vi "Curtin1_NotesDialog.vi"(11 "Files":T1[](array[typedef])) -> (0 "Color":u32[](array[colorbox]), 2 "removed?":bool, 3 "Array":T1[](array[typedef]))   [LabVIEW 2022 SP3]
uses:
  Curtin1_Label.ctl
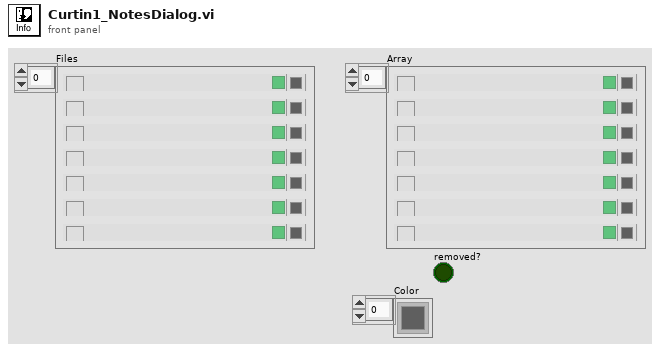
[diagram p1: front panel]
types:
  T1 = typedef "Curtin1_Label.ctl" = cluster{"Show?":bool, "Name":string, "Color":u32, "Path":path, "Show Notes":bool, "correlate":bool}
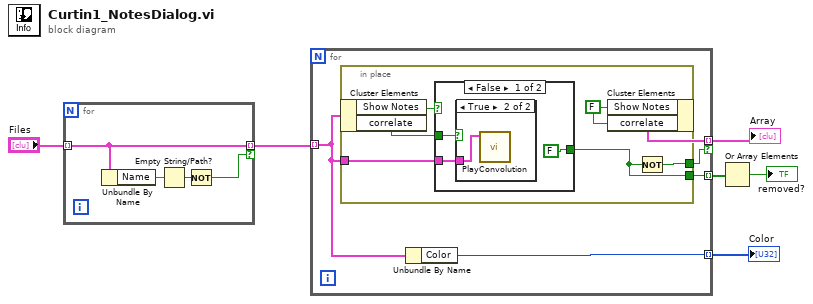
[diagram p0: block diagram]
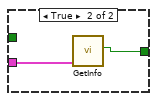
[diagram p3: hidden frame]
diagram:
  n1 = for {
    tunnel: "Files" -> [w9] mode=indexing
    tunnel: [w9] -> w3 mode=indexing if=w7
    n2 = Unbundle By Name(w9) -> ("Name"=w10:string)
    n3 = Empty String/Path?(string/path=w10) -> (empty?=w8:bool)
    n4 = Not(x=w8) -> (.not. x?=w7:bool)
  }
  n5 = for {
    tunnel: w3 -> [w14] mode=indexing
    tunnel: [w15] -> w6 mode=indexing if=w12
    tunnel: [w13] -> w5 mode=indexing
    tunnel: [w11] -> w2 mode=indexing
    n6 = in-place {
      in-place-border: w14 -> [w20]
      in-place-border: [w19] -> w12
      in-place-border: [w18] -> w11
      w17 = FALSE ("Show Notes")
      n7 = in-place-cluster #1(w14) -> ("Show Notes"=w21:bool, "correlate"=w16:bool)
      n8 = case shown="False" w21 {
        tunnel: w20 -> [w22 w27]
        tunnel: [FALSE ("remove?") w26] -> w18
        tunnel: w16 -> [w23 _]
        frame False {
          n9 = case shown="True" w23 {
            tunnel: w22 -> [_ w25]
            frame False {
            }
            frame True {
              n10 = call "PlayConvolution.vi"("File"=w25) -> ()  [unwired: 11 in]
            }
          }
        }
        frame True {
          n11 = call "GetInfo.vi"("File selected"=w27) -> ("remove?"=w26:bool)  [unwired: 10 in]
        }
      }
      n12 = in-place-cluster #1("Show Notes"=w17, "correlate"=w17) -> (w15:T1)
      n13 = Not(x=w18) -> (.not. x?=w19:bool)
    }
    n14 = Unbundle By Name(w14) -> ("Color"=w13:u32)
  }
  "Array" <- w6
  "Color" <- w5
  n15 = Or Array Elements(Boolean array=w2) -> (logical OR=→"removed?":bool)
